vi "EjemploPrueba.vi"(3 "Original":T1) -> (0 "AreaHerida":dbl, 1 "Mask":T1)   [LabVIEW 2021]
uses:
  <vilib>/vision/Image Controls.llb/IMAQ Image.ctl
  <vilib>/Utility/file.llb/Read Delimited Spreadsheet (string).vi
  <vilib>/vision/NI_Vision_Development_Module.lvlib
panel:
  out "all rows":string[][](array[string])
  out "Masky":T1(plugin-control)
  out "Originaly":T1(plugin-control)
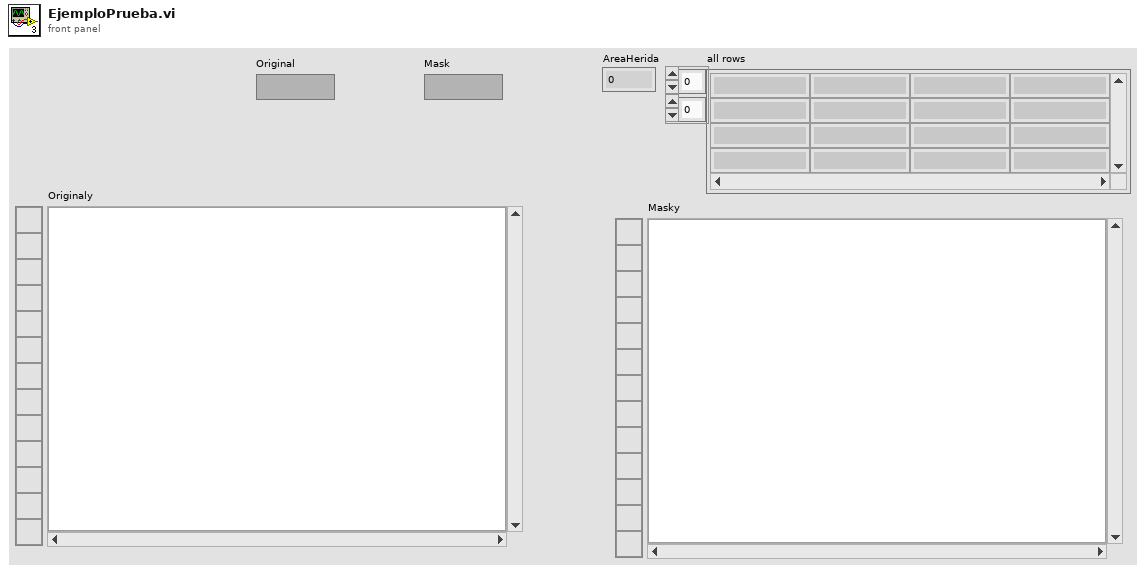
[diagram p1: front panel]
types:
  T1 = typedef "IMAQ Image.ctl" = refnum<image>
  T2 = typedef "Particle Parameters" = i32
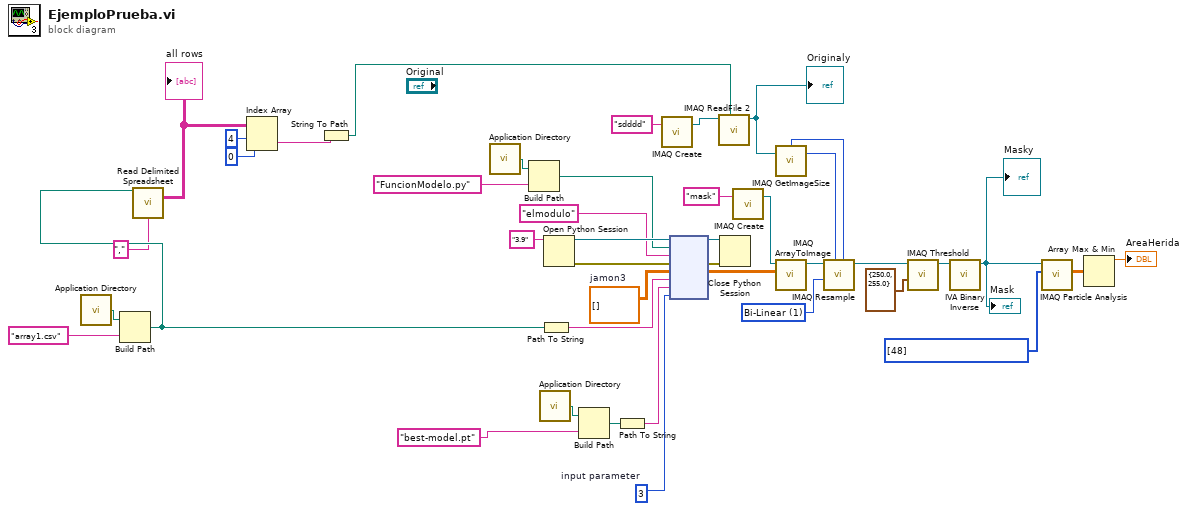
[diagram p0: block diagram]
diagram:
  w8 = 3  # input parameter
  w18 = T2[] [48] items=["Center of Mass X", "Center of Mass Y", "First Pixel X", "First Pixel Y", "Bounding Rect Left", "Bounding Rect Top", "Bounding Rect Right", "Bounding Rect Bottom", "Max Feret Diameter Start X", "Max Feret Diameter Start Y", "Max Feret Diameter End X", "Max Feret Diameter End Y", "Max Horiz. Segment Length Left", "Max Horiz. Segment Length Right", "Max Horiz. Segment Length Row", "-", "Bounding Rect Width", "Bounding Rect Height", "Bounding Rect Diagonal", "Perimeter", "Convex Hull Perimeter", "Holes' Perimeter", "Max Feret Diameter", "Equivalent Ellipse Major Axis", "Equivalent Ellipse Minor Axis", "Equivalent Ellipse Minor Axis (Feret)", "Equivalent Rect Long Side", "Equivalent Rect Short Side", "Equivalent Rect Diagonal", "Equivalent Rect Short Side (Feret)", "Average Horiz. Segment Length", "Average Vert. Segment Length", "Hydraulic Radius", "Waddel Disk Diameter", "-", "Area", "Holes' Area", "Particle & Holes' Area", "Convex Hull Area", "Image Area", "-", "Number of Holes", "Number of Horiz. Segments", "Number of Vert. Segments", "-", "Orientation", "Max Feret Diameter Orientation", "-", "% Area/Image Area", "% Area/(Particle & Holes' Area)", "Ratio of Equivalent Ellipse Axes", "Ratio of Equivalent Rect Sides", "-", "Elongation Factor", "Compactness Factor", "Heywood Circularity Factor", "Type Factor", "-", "Sum X", "Sum Y", "Sum XX", "Sum XY", "Sum YY", "Sum XXX", "Sum XXY", "Sum XYY", "Sum YYY", "-", "Moment of Inertia XX", "Moment of Inertia XY", "Moment of Inertia YY", "Moment of Inertia XXX", "Moment of Inertia XXY", "Moment of Inertia XYY", "Moment of Inertia YYY", "Norm. Moment of Inertia XX", "Norm. Moment of Inertia XY", "Norm. Moment of Inertia YY", "Norm. Moment of Inertia XXX", "Norm. Moment of Inertia XXY", "Norm. Moment of Inertia XYY", "Norm. Moment of Inertia YYY", "Hu Moment 1", "Hu Moment 2", "Hu Moment 3", "Hu Moment 4", "Hu Moment 5", "Hu Moment 6", "Hu Moment 7"] ("Pixel Measurements")
  w33 = u32 1 items=["Zero Order", "Bi-Linear", "Quadratic", "Cubic Spline"] ("Interpolation Type")
  w37 = dbl[][] []  # jamon3
  n1 = call <vilib>:"Application Directory.vi"() -> ("Application Directory"=w23:path)
  n2 = Build Path(base path=w23, name or relative path="array1.csv") -> (appended path=w7:path)
  n3 = call-poly <vilib>:"Read Delimited Spreadsheet.vi"("file path (dialog if empty)"=w7, "delimiter (\\t)"="," ("delimiter (\\t)")) -> ("all rows"=w5:string[][])  [unwired: 8 in, 5 out]
  "all rows" <- w5
  n4 = Index Array(array=w5, index (row)=4, index (col)=0 ("disabled index (col)")) -> (element=w6:string)
  n5 = String To Path(string=w6) -> (path=w2:path)
  n6 = call <vilib>:"Application Directory.vi"() -> ("Application Directory"=w21:path)
  n7 = Build Path(base path=w21, name or relative path="FuncionModelo.py") -> (appended path=w20:path)
  n8 = call <vilib>:"Application Directory.vi"() -> ("Application Directory"=w26:path)
  n9 = Path To String(path=w7) -> (string=w28:string)
  n10 = Open Python Session(python version="3.9" ("Python version")) -> (session out=w42:refnum<k35>, error out=w40:errorcluster)  [unwired: 2 in]
  n11 = Build Path(base path=w26, name or relative path="best-model.pt") -> (appended path=w25:path)
  n12 = Path To String(path=w25) -> (string=w27:string)
  n13 = call "IMAQ Create"("Image Name"="sdddd") -> ("New Image"=w12:T1)  [unwired: 4 in, 1 out]
  n14 = node(w42, w20, "elmodulo" ("function name"), w40, w37, w28, w27, w8) -> (w41:refnum<k35>, w39:errorcluster, w36:dbl[][])  [unwired: 3 in, 2 out]
  n15 = call "IMAQ ReadFile 2"("File Path"=w2, "Image"=w12) -> ("Image Out"=w10:T1)  [unwired: 5 in, 4 out]
  "Originaly" <- w10
  n16 = Close Python Session(session in=w41, error in=w39) -> ()  [unwired: 1 out]
  n17 = call "IMAQ Create"("Image Name"="mask") -> ("New Image"=w35:T1)  [unwired: 4 in, 1 out]
  n18 = call "IMAQ GetImageSize"("Image"=w10) -> ("Y Resolution"=w31:i32, "X Resolution"=w30:i32)  [unwired: 3 in, 1 out]
  n19 = call "IMAQ ArrayToImage"("Image Pixels (U8)"=w36, "Image"=w35) -> ("Image Out"=w29:T1)  [unwired: 8 in, 1 out]
  n20 = call "IMAQ Resample"("X Resolution"=w30, "Y Resolution"=w31, "Interpolation Type"=w33, "Image Src"=w29) -> ("Image Dst Out"=w14:T1)  [unwired: 6 in, 1 out]
  n21 = call "IMAQ Threshold"("Range"=cluster{"Lower value":sgl, "Upper value":sgl} {"Lower value"=250.0, "Upper value"=255.0}, "Image Src"=w14) -> ("Image Dst Out"=w19:T1)  [unwired: 8 in, 1 out]
  n22 = call <vilib>:"IVA Binary Inverse.vi"("Image In"=w19) -> ("Image Out"=w13:T1)  [unwired: 1 in, 9 out]
  "Mask" <- w13
  "Masky" <- w13
  n23 = call "IMAQ Particle Analysis"("Pixel Measurements"=w18, "Image"=w13) -> ("Particle Measurements (Pixels)"=w17:dbl[][])  [unwired: 4 in, 5 out]
  n24 = Array Max & Min(array=w17) -> (max value=→"AreaHerida":dbl)  [unwired: 3 out]
